vi "Heat Up Macro Search Previous.vi"(8 "Error In":errorcluster, 10 "Step 8":string[][](array[string]), 11 "Step 7":string[][](array[string])) -> (0 "Error Out":errorcluster, 1 "index of element 2":i32, 2 "Array 2":i32[](array[numeric]), 3 "size(s)":i32[](array[numeric]), 4 "subarray":string[][](array[string]), 5 "Array":string[][](array[string]), 6 "Output Array":string[][](array[string]), 7 "index of element":i32)   [LabVIEW 2019]
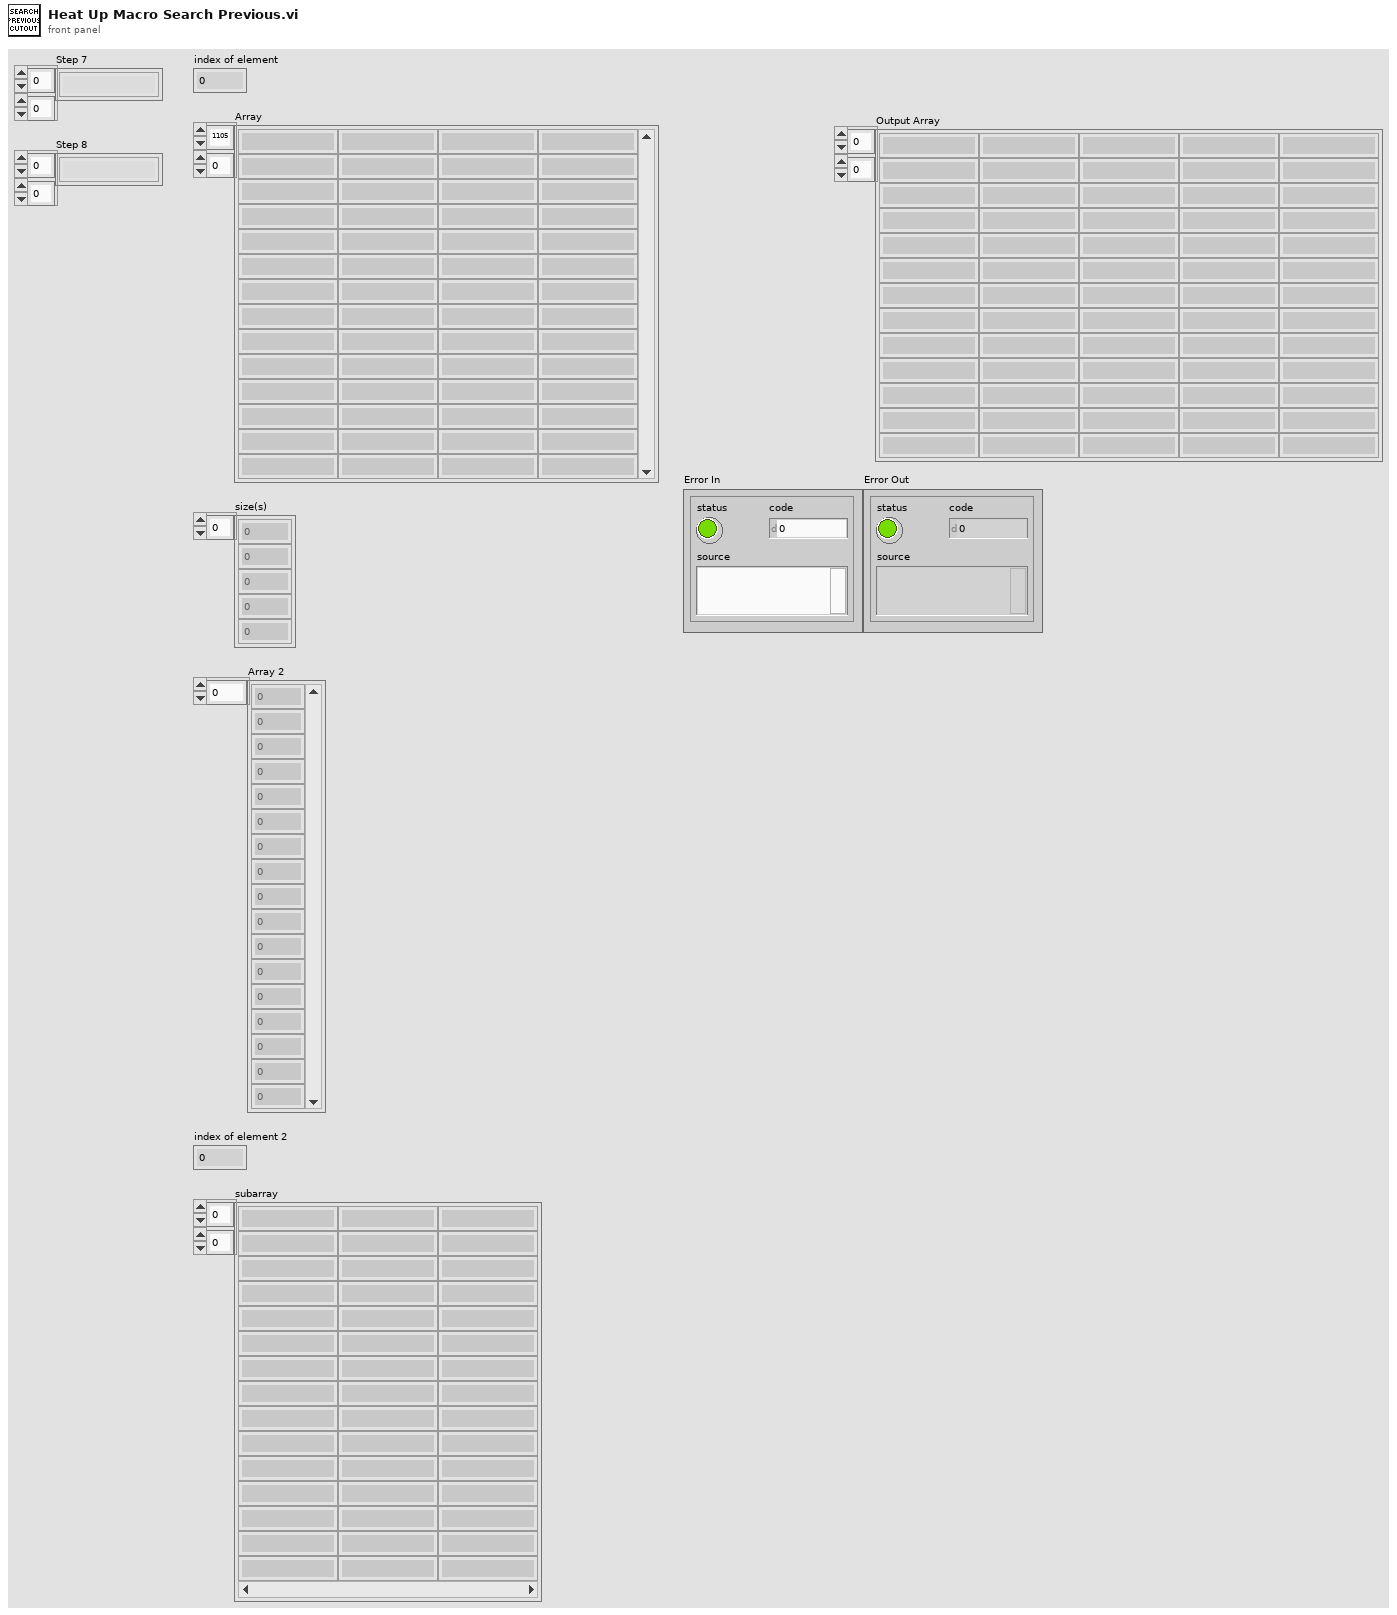
[diagram p1: front panel]
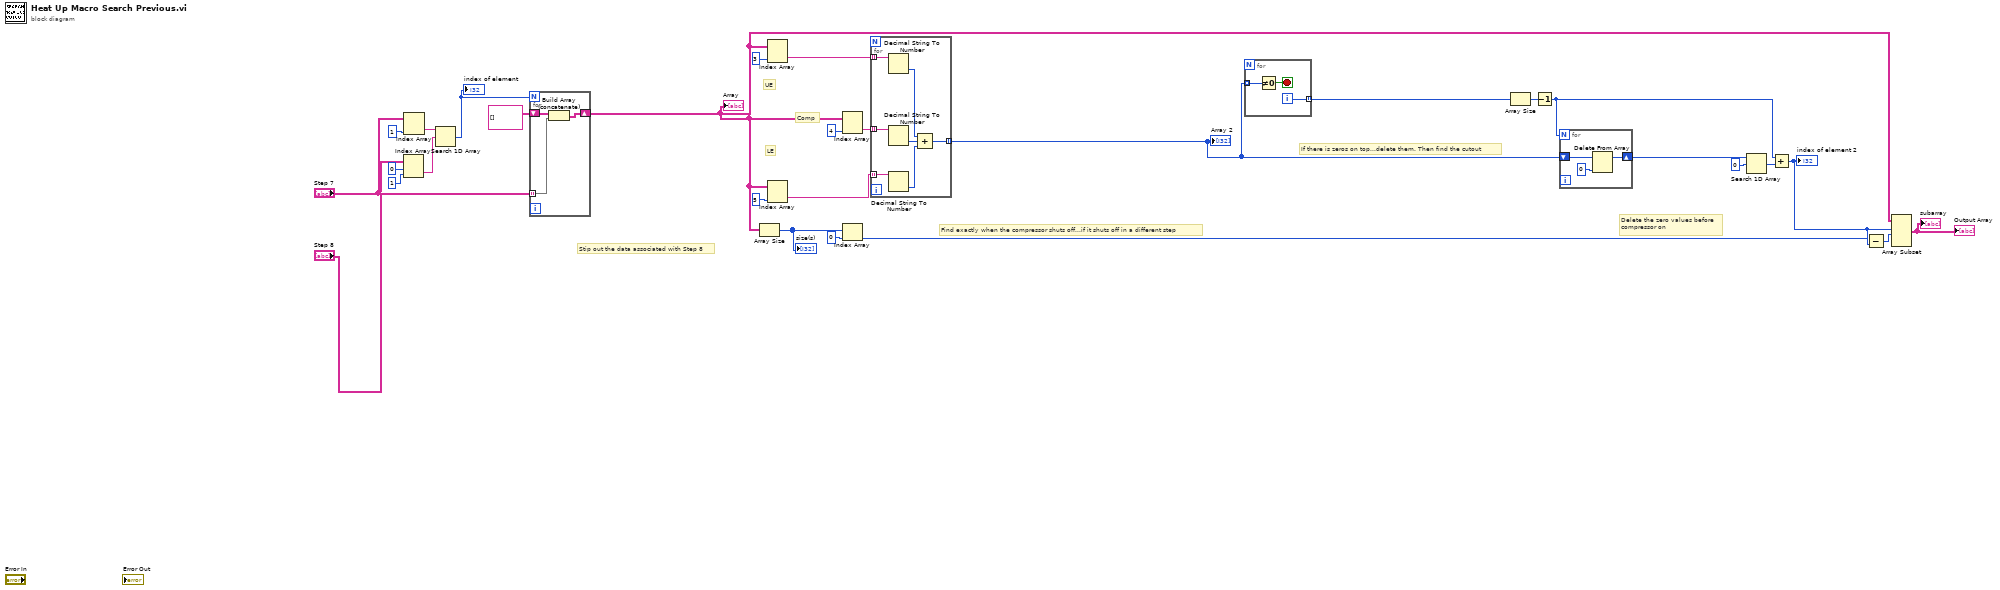
[diagram p0: block diagram]
diagram:
  # "Delete the zero values before \ncompressor on"
  # "If there is zeros on top...delete them. Then find the cutout"
  # "Comp"
  # "LE"
  # "UE"
  # "Find exactly when the compressor shuts off...if it shuts off in a different step"
  # "Stip out the data associated with Step 8"
  n1 = Index Array(array="Step 8", index (row)=0 ("disabled index (row)"), index (col)=1 ("disabled index (col)")) -> (element=w5:string)
  n2 = Index Array(array="Step 7", index (col)=1 ("disabled index (col)")) -> (element=w4:string[])  [unwired: 1 in]
  n3 = Search 1D Array(1D array=w4, element=w5) -> (index of element=w7:i32)  [unwired: 1 in]
  "index of element" <- w7
  n4 = for {
    N: w7 -> [_]
    shift-right: [w31] -> w17
    shift-left: string[][] [] -> [w32]
    tunnel: "Step 7" -> [w30] mode=indexing
    n5 = Build Array (concatenate)(w32, w30) -> (w31:string[][])
  }
  "Array" <- w17
  n6 = Array Size(array=w17) -> (size(s)=w15:i32[])
  "size(s)" <- w15
  n7 = Index Array(array=w17, index (col)=3 ("disabled index (col)")) -> (element=w14:string[])  [unwired: 1 in]
  n8 = Index Array(array=w17, index (col)=5 ("disabled index (col)")) -> (element=w13:string[])  [unwired: 1 in]
  n9 = Index Array(array=w17, index (col)=4 ("disabled index (col)")) -> (element=w9:string[])  [unwired: 1 in]
  n10 = Index Array(array=w15, index=0) -> (element=w18:i32)
  n11 = for {
    tunnel: w9 -> [w39] mode=indexing
    tunnel: w13 -> [w38] mode=indexing
    tunnel: w14 -> [w37] mode=indexing
    tunnel: [w33] -> w24 mode=indexing
    n12 = Decimal String To Number(string=w37) -> (number=w36:i32)  [unwired: 2 in, 1 out]
    n13 = Decimal String To Number(string=w39) -> (number=w35:i32)  [unwired: 2 in, 1 out]
    n14 = Decimal String To Number(string=w38) -> (number=w34:i32)  [unwired: 2 in, 1 out]
    n15 = Compound Arithmetic op=ADD(w36, w35, w34) -> (w33:i32)
  }
  "Array 2" <- w24
  n16 = for {
    tunnel: w24 -> [w42] mode=indexing
    tunnel: [w40] -> w22 mode=indexing
    i -> [w40]
    stop <- w41 stop-if-true
    n17 = Not Equal To 0?(x=w42) -> (x != 0?=w41:bool)
  }
  n18 = Array Size(array=w22) -> (size(s)=w23:i32)
  n19 = Decrement(x=w23) -> (x-1=w28:i32)
  n20 = for {
    N: w28 -> [_]
    shift-right: [w43] -> w25
    shift-left: w24 -> [w45]
    n21 = Delete From Array(array=w45, index=0) -> (array with subset deleted=w43:i32[])  [unwired: 1 in, 1 out]
  }
  n22 = Search 1D Array(1D array=w25, element=0) -> (index of element=w26:i32)  [unwired: 1 in]
  n23 = Add(x=w28, y=w26) -> (x+y=w27:i32)
  "index of element 2" <- w27
  n24 = Subtract(x=w18, y=w27) -> (x-y=w19:i32)
  n25 = Array Subset(array=w17, index (row)=w27, length (row)=w19) -> (→"subarray" →"Output Array":string[][])  [unwired: 2 in]
